vi "Vision Aim 359 - AUTO.vi"(11 "abort":bool) -> (0 "ARM GOOD":bool, 1 "WHEELS GOOD":bool, 2 "Vision In Range?":bool, 3 "Gyro":dbl=-7.62231046031169 format="%.2f", 4 "Vision Tolerance  Out":dbl=0.05)   [LabVIEW 2015]
uses:
  <vilib>/addons/control/pid/pid.llb/PID Control Input Filter (DBL).vi
  Code/Robot Global Data.vi
  <vilib>/Rock Robotics/WPI/Utilities/WPI_GetSetVariantRefNum.vi
  <vilib>/Rock Robotics/WPI/RobotDrive/WPI_RobotDriveArcadeDrive_Standard(NoSaturation).vi
  <vilib>/addons/control/pid/NI_PID_pid.lvlib
panel:
  out "Enum":T1(ring)=enum."Stop"
  out "Vision":dbl=0.057812500000000086 format="%.2f"
  in  "Range 2":dbl=0.03
  in  "Speed 2":dbl=0.35
  in  "Speed 1":dbl=0.55
  in  "Range 1":dbl=0.2
  in  "Vision Tolerance":dbl=0.05
  # "Outputs"
  # "Turning Gains"
  # ".5"
  # ".4 pg"
  # ".45"
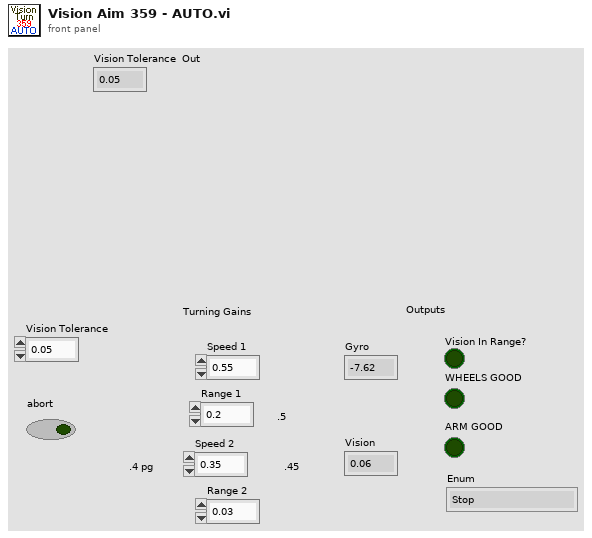
[diagram p1: front panel]
types:
  T1 = enum16{"Init", "Turn Coarse", "Turn Fine ", "Shoot?", "Stop", "Done"}
  T2 = enum16{"Init", "Turn Coarse", "Turn Fine ", "Shoot?", "Stop"}
  T3 = typedef "WPI_RobotDriveDevRef.ctl" = cluster{"DevStatus":errorcluster, "Motors[]":T4[], "Square Inputs":bool, "Max Output":dbl}
  T4 = typedef "WPI_MotorControlDeviceRef.ctl" = cluster{"DeviceStatus":errorcluster, "Type":T5, "PWM":cluster{"PWM Channel":T6, "DeadBand":T7}, "CAN":cluster{"Device Number":u8, "Control Mode":T8, "Semaphore":T9, "Max Vout":dbl, "TalonSRX Control Mode":T10}, "Invert":bool}
  T5 = typedef "WPI_MotorControlType.ctl" = enum16{"PWM", "CAN", "CANTalonSRX"}
  T6 = typedef "FPGA_DIOPWMChannel.ctl" = enum8{"PWM 0", "PWM 1", "PWM 2", "PWM 3", "PWM 4", "PWM 5", "PWM 6", "PWM 7", "PWM 8", "PWM 9", "PWM MXP 0", "PWM MXP 1", "PWM MXP 2", "PWM MXP 3", "PWM MXP 4", "PWM MXP 5", "PWM MXP 6", "PWM MXP 7", "PWM MXP 8", "PWM MXP 9", "Invalid"}
  T7 = typedef "WPI_PWMDeadband.ctl" = cluster{"Name":string, "maxPositivePwm":i32, "minPositivePwm":i32, "centerPwm":i32, "maxNegativePwm":i32, "minNegativePwm":i32, "angularRange":u16}
  T8 = typedef "WPI_CANJaguar_ControlMode.ctl" = enum8{"Percent VBus", "Current", "Speed", "Position", "Voltage"}
  T9 = typedef "Semaphore RefNum" = refnum<k1>
  T10 = typedef "WPI_CANTalonSRX_APIControlMode.ctl" = enum8{"Percent VBus", "Speed", "Position", "Slave", "Unchanged / Invalid", "Voltage Compensation", "Current", "Motion Profile"}
  T11 = typedef "WPI_GyroDevRef.ctl" = cluster{"DevStatus":errorcluster, "Analog Channel":T12, "Offset":dbl, "Gain (VoltsPerDegree/Second)":dbl, "Gyro Type":enum16{"Analog", "XRS450"}, "Handle":i32, "SPI Bus":T13, "Device Found":bool, "Sample Rate":dbl, "Calibrate On Open":bool}
  T12 = typedef "FPGA_AIChannel.ctl" = enum8{"AI 0", "AI 1", "AI 2", "AI 3", "AI MXP 0", "AI MXP 1", "AI MXP 2", "AI MXP 3", "Invalid"}
  T13 = typedef "spi_bus.ctl" = enum16{"SPI On-Board, CS0", "SPI On-Board, CS1", "SPI On-Board, CS2", "SPI On-Board, CS3", "SPI MXP", "Invalid"}
  T14 = enum16{"Init", "Get Angle", "Turn Angle ", "Shoot?", "Stop"}
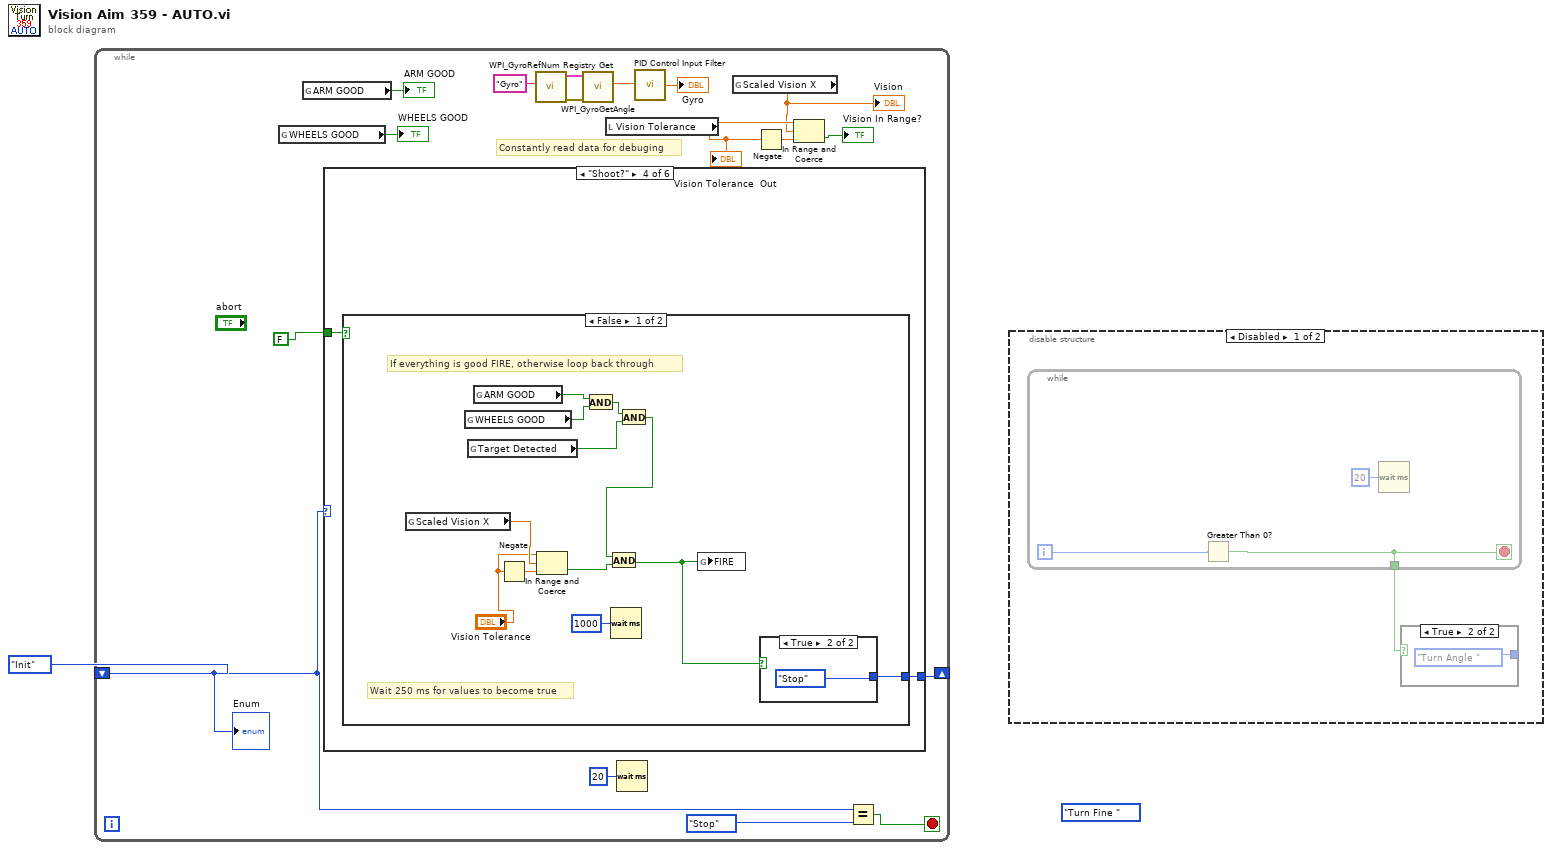
[diagram p0: block diagram]
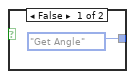
[diagram p2: hidden frame]
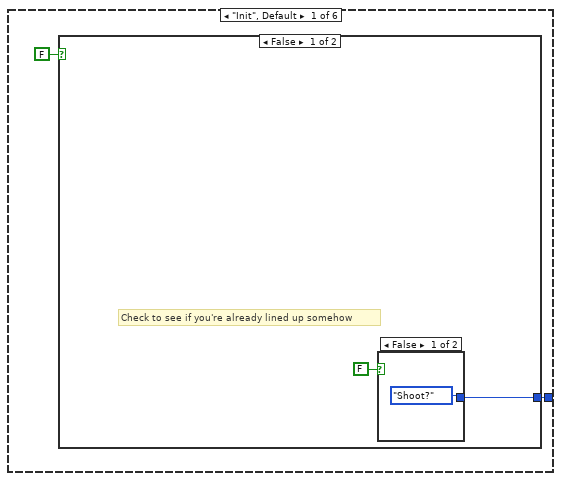
[diagram p4: hidden frame]
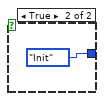
[diagram p5: hidden frame]
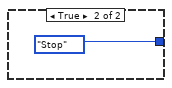
[diagram p6: hidden frame]
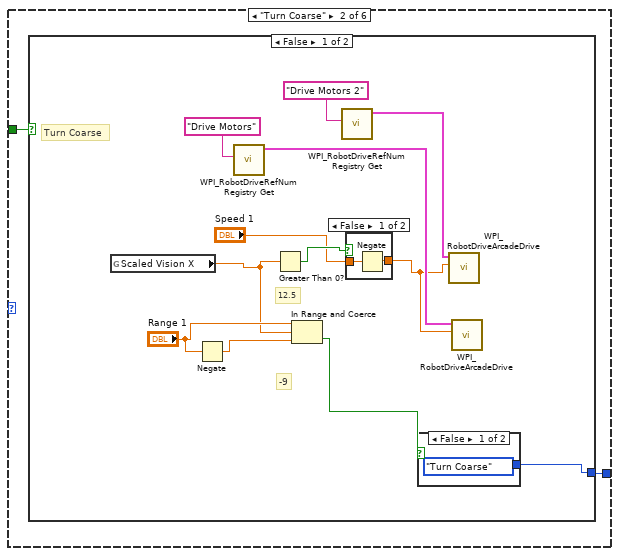
[diagram p7: hidden frame]
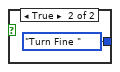
[diagram p8: hidden frame]
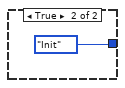
[diagram p10: hidden frame]
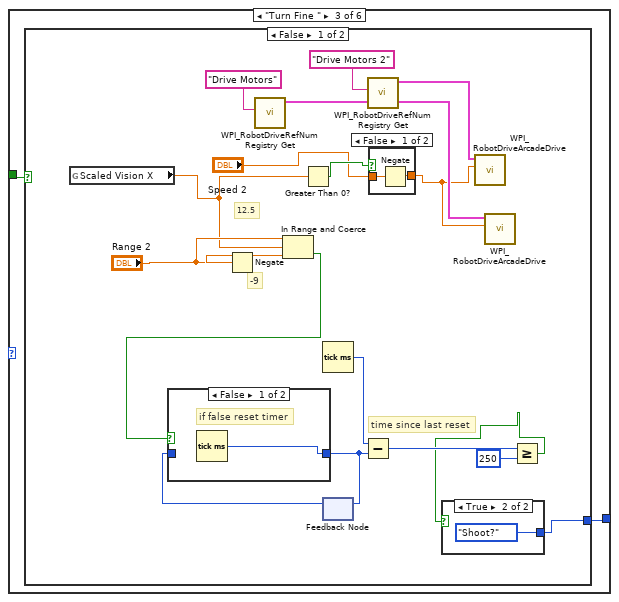
[diagram p11: hidden frame]
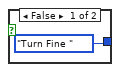
[diagram p12: hidden frame]
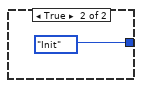
[diagram p15: hidden frame]
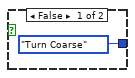
[diagram p16: hidden frame]
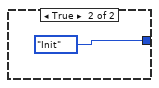
[diagram p17: hidden frame]
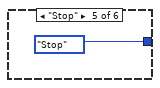
[diagram p18: hidden frame]
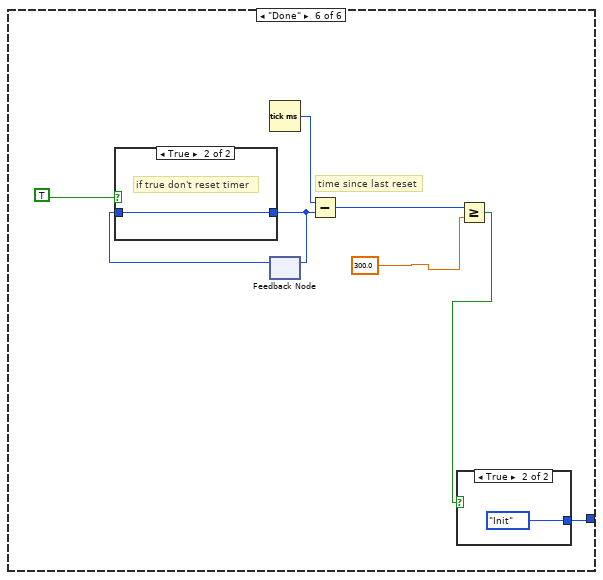
[diagram p19: hidden frame]
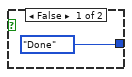
[diagram p20: hidden frame]
diagram:
  (unwired) T2."Turn Fine "
  n1 = while {
    shift-right: [w18] -> _
    shift-left: T1."Init" -> [w16]
    stop <- w17 stop-if-true
    # "Constantly read data for debuging"
    n2 = global read "Robot Global Data.vi" "WHEELS GOOD"() -> (→"WHEELS GOOD":bool)
    n3 = global read "Robot Global Data.vi" "ARM GOOD"() -> (→"ARM GOOD":bool)
    n4 = case shown="\"Shoot?\"" w16 {
      tunnel: [w20 w27 w47 w75 T2."Stop" w93] -> w18
      tunnel: FALSE -> [_ w26 w46 w74 _ _]
      frame "Init", Default {
        n5 = case shown="False" FALSE {
          tunnel: [w22 T2."Stop"] -> w20
          frame False {
            # "Check to see if you're already lined up somehow"
            n6 = case shown="False" FALSE {
              tunnel: [T1."Shoot?" T1."Init"] -> w22
              frame False {
              }
              frame True {
              }
            }
          }
          frame True {
          }
        }
      }
      frame "Turn Coarse" {
        n7 = case shown="False" w26 {
          tunnel: [w35 T2."Init"] -> w27
          frame False {
            # "-9"
            # "12.5"
            # "Turn Coarse"
            n8 = global read "Robot Global Data.vi" "Scaled Vision X"() -> (w30:dbl)
            n9 = Negate(x="Range 1") -> (-x=w32:dbl)
            n10 = call <vilib>:"WPI_RobotDriveRefNum Registry Get.vi"("refnum name"="Drive Motors") -> ("RobotDriveDevRef"=w38:T3)  [unwired: 1 in, 9 out]
            n11 = Greater Than 0?(x=w30) -> (x > 0?=w34:bool)
            n12 = In Range and Coerce(upper limit="Range 1", x=w30, lower limit=w32) -> (In Range?=w28:bool)  [unwired: 1 out]
            n13 = call <vilib>:"WPI_RobotDriveRefNum Registry Get.vi"("refnum name"="Drive Motors 2") -> ("RobotDriveDevRef"=w36:T3)  [unwired: 1 in, 9 out]
            n14 = case shown="False" w34 {
              tunnel: "Speed 1" -> [w43 w44]
              tunnel: [w42 w44] -> w29
              frame False {
                n15 = Negate(x=w43) -> (-x=w42:dbl)
              }
              frame True {
              }
            }
            n16 = case shown="False" w28 {
              tunnel: [T2."Turn Coarse" T2."Turn Fine "] -> w35
              frame False {
              }
              frame True {
              }
            }
            n17 = call-poly <vilib>:"WPI_RobotDriveArcadeDrive.vi"("X axis value"=w29, "RobotDriveDevRef"=w36) -> ()  [unwired: 7 in, 3 out]
            n18 = call-poly <vilib>:"WPI_RobotDriveArcadeDrive.vi"("X axis value"=w29, "RobotDriveDevRef"=w38) -> ()  [unwired: 7 in, 3 out]
          }
          frame True {
          }
        }
      }
      frame "Turn Fine " {
        n19 = case shown="False" w46 {
          tunnel: [w61 T2."Init"] -> w47
          frame False {
            # "time since last reset"
            # "-9"
            # "12.5"
            n20 = global read "Robot Global Data.vi" "Scaled Vision X"() -> (w56:dbl)
            n21 = Negate(x="Range 2") -> (-x=w59:dbl)
            n22 = call <vilib>:"WPI_RobotDriveRefNum Registry Get.vi"("refnum name"="Drive Motors") -> ("RobotDriveDevRef"=w62:T3)  [unwired: 1 in, 9 out]
            n23 = In Range and Coerce(upper limit="Range 2", x=w56, lower limit=w59) -> (In Range?=w50:bool)  [unwired: 1 out]
            n24 = Greater Than 0?(x=w56) -> (x > 0?=w60:bool)
            n25 = Tick Count (ms)() -> (millisecond timer value=w54:u32)
            n26 = feedback #1() -> (w53:u32)  [unwired: 1 in]
            n27 = case shown="False" w50 {
              tunnel: [w68 w69] -> w52
              tunnel: w53 -> [_ w69]
              frame False {
                # "if false reset timer"
                n28 = Tick Count (ms)() -> (millisecond timer value=w68:u32)
              }
              frame True {
                # "if true don't reset timer"
              }
            }
            n29 = feedback-in #1(w52) -> ()
            n30 = Subtract(x=w54, y=w52) -> (x-y=w51:u32)
            n31 = call <vilib>:"WPI_RobotDriveRefNum Registry Get.vi"("refnum name"="Drive Motors 2") -> ("RobotDriveDevRef"=w63:T3)  [unwired: 1 in, 9 out]
            n32 = case shown="False" w60 {
              tunnel: "Speed 2" -> [w71 w72]
              tunnel: [w70 w72] -> w55
              frame False {
                n33 = Negate(x=w71) -> (-x=w70:dbl)
              }
              frame True {
              }
            }
            n34 = call-poly <vilib>:"WPI_RobotDriveArcadeDrive.vi"("X axis value"=w55, "RobotDriveDevRef"=w63) -> ()  [unwired: 7 in, 3 out]
            n35 = call-poly <vilib>:"WPI_RobotDriveArcadeDrive.vi"("X axis value"=w55, "RobotDriveDevRef"=w62) -> ()  [unwired: 7 in, 3 out]
            n36 = Greater Or Equal?(x=w51, y=u32 250) -> (x >= y?=w48:bool)
            n37 = case shown="True" w48 {
              tunnel: [T2."Turn Fine " T2."Shoot?"] -> w61
              frame False {
              }
              frame True {
              }
            }
          }
          frame True {
          }
        }
      }
      frame "Shoot?" {
        n38 = case shown="False" w74 {
          tunnel: [w87 T2."Init"] -> w75
          frame False {
            # "Wait 250 ms for values to become true"
            # "If everything is good FIRE, otherwise loop back through"
            n39 = global read "Robot Global Data.vi" "Scaled Vision X"() -> (w83:dbl)
            n40 = global read "Robot Global Data.vi" "WHEELS GOOD"() -> (w84:bool)
            n41 = global read "Robot Global Data.vi" "Target Detected"() -> (w77:bool)
            n42 = global read "Robot Global Data.vi" "ARM GOOD"() -> (w85:bool)
            n43 = Negate(x="Vision Tolerance") -> (-x=w81:dbl)
            n44 = In Range and Coerce(upper limit="Vision Tolerance", x=w83, lower limit=w81) -> (In Range?=w86:bool)  [unwired: 1 out]
            n45 = And(x=w85, y=w84) -> (x .and. y?=w78:bool)
            n46 = Wait (ms)(milliseconds to wait=u32 1000) -> ()  [unwired: 1 out]
            n47 = And(x=w78, y=w77) -> (x .and. y?=w76:bool)
            n48 = And(x=w76, y=w86) -> (x .and. y?=w79:bool)
            n49 = global write "Robot Global Data.vi" "FIRE"(w79) -> ()
            n50 = case shown="True" w79 {
              tunnel: [T2."Turn Coarse" T1."Stop"] -> w87
              frame False {
              }
              frame True {
              }
            }
          }
          frame True {
          }
        }
      }
      frame "Stop" {
      }
      frame "Done" {
        # "time since last reset"
        n51 = Tick Count (ms)() -> (millisecond timer value=w95:u32)
        n52 = feedback #2() -> (w98:u32)  [unwired: 1 in]
        n53 = case shown="True" TRUE {
          tunnel: [w102 w103] -> w96
          tunnel: w98 -> [_ w103]
          frame False {
            # "if false reset timer"
            n54 = Tick Count (ms)() -> (millisecond timer value=w102:u32)
          }
          frame True {
            # "if true don't reset timer"
          }
        }
        n55 = feedback-in #2(w96) -> ()
        n56 = Subtract(x=w95, y=w96) -> (x-y=w97:u32)
        n57 = Greater Or Equal?(x=w97, y=300.0 ("Delay (ms)")) -> (x >= y?=w92:bool)
        n58 = case shown="True" w92 {
          tunnel: [T1."Done" T1."Init"] -> w93
          frame False {
          }
          frame True {
          }
        }
      }
    }
    n59 = call <vilib>:"WPI_GyroRefNum Registry Get.vi"("refnum name"="Gyro") -> ("error out"=w8:errorcluster, "GyroDevRef"=w7:T11)  [unwired: 9 in]
    n60 = call <vilib>:"WPI_GyroGetAngle.vi"("error in"=w8, "GyroDevRef"=w7) -> ("Angle"=w6:dbl)  [unwired: 5 in, 4 out]
    n61 = local read "Vision Tolerance"() -> (w14:dbl)
    "Vision Tolerance  Out" <- w14
    n62 = Wait (ms)(milliseconds to wait=u32 20) -> ()  [unwired: 1 out]
    n63 = call-poly <vilib>:"PID Control Input Filter.vi"("input"=w6) -> ("output"=→"Gyro":dbl)  [unwired: 4 in]
    n64 = global read "Robot Global Data.vi" "Scaled Vision X"() -> (w3:dbl)
    "Vision" <- w3
    n65 = Negate(x=w14) -> (-x=w13:dbl)
    n66 = In Range and Coerce(upper limit=w14, x=w3, lower limit=w13) -> (In Range?=→"Vision In Range?":bool)  [unwired: 1 out]
    n67 = Equal?(x=w16, y=T2."Stop") -> (x = y?=w17:bool)
    "Enum" <- w16
  }
  n68 = disable-structure shown="Disabled" {
    frame Disabled {
      n69 = while {
        tunnel: [w109] -> w104
        i -> [w108]
        stop <- w109 stop-if-true
        n70 = Greater Than 0?(x=w108) -> (x > 0?=w109:bool)
        n71 = Wait (ms)(milliseconds to wait=u32 20) -> ()  [unwired: 1 out]
      }
      n72 = case shown="True" w104 {
        tunnel: [T14."Get Angle" T14."Turn Angle "] -> _
        frame False {
        }
        frame True {
        }
      }
    }
    frame Enabled {
    }
  }
